vi "DV_Adjust_Histogram_Cursor.vi"(10 "lock to bin edges":bool, 11 "histogram reference":refnum<vi>) -> ()   [LabVIEW 2016]
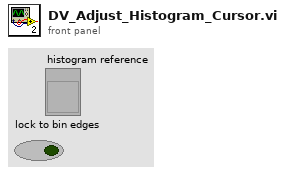
[diagram p1: front panel]
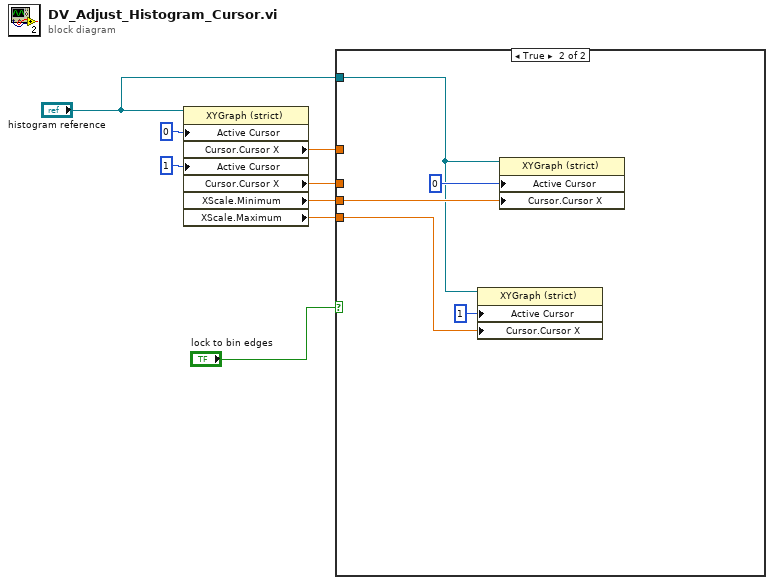
[diagram p0: block diagram]
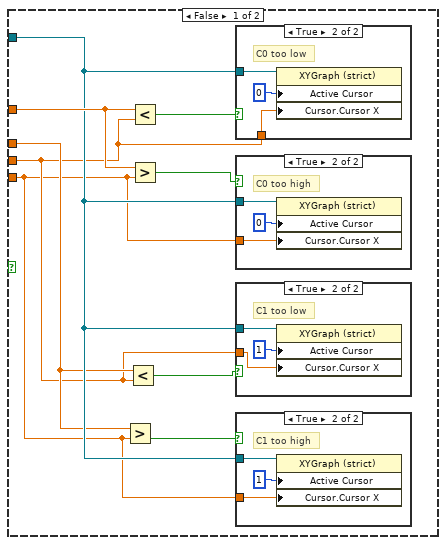
[diagram p2: hidden frame]
diagram:
  n1 = property on="Property Node" class="XYGraph (strict)"(reference="histogram reference", "Active Cursor"=0, "Active Cursor"=1) -> ("Cursor.Cursor X"=w6:dbl, "Cursor.Cursor X"=w4:dbl, "XScale.Minimum"=w3:dbl, "XScale.Maximum"=w2:dbl)  [unwired: 1 in, 2 out]
  n2 = case shown="True" "lock to bin edges" {
    tunnel: w6 -> [w16 _]
    tunnel: "histogram reference" -> [w14 w30]
    tunnel: w4 -> [w11 _]
    tunnel: w3 -> [w10 w33]
    tunnel: w2 -> [w9 w31]
    frame False {
      n3 = Greater?(x=w11, y=w9) -> (0:w12:bool)
      n4 = Less?(x=w11, y=w10) -> (x < y?=w13:bool)
      n5 = Less?(x=w16, y=w10) -> (x < y?=w17:bool)
      n6 = Greater?(x=w16, y=w9) -> (0:w15:bool)
      n7 = case shown="True" w17 {
        tunnel: w14 -> [_ w28]
        tunnel: w10 -> [_ w27]
        frame False {
        }
        frame True {
          # "C0 too low"
          n8 = property on="Property Node" class="XYGraph (strict)"(reference=w28, "Active Cursor"=0, "Cursor.Cursor X"=w27) -> ()  [unwired: 1 in, 2 out]
        }
      }
      n9 = case shown="True" w15 {
        tunnel: w14 -> [_ w25]
        tunnel: w9 -> [_ w24]
        frame False {
        }
        frame True {
          # "C0 too high"
          n10 = property on="Property Node" class="XYGraph (strict)"(reference=w25, "Active Cursor"=0, "Cursor.Cursor X"=w24) -> ()  [unwired: 1 in, 2 out]
        }
      }
      n11 = case shown="True" w13 {
        tunnel: w14 -> [_ w22]
        tunnel: w10 -> [_ w21]
        frame False {
        }
        frame True {
          # "C1 too low"
          n12 = property on="Property Node" class="XYGraph (strict)"(reference=w22, "Active Cursor"=1, "Cursor.Cursor X"=w21) -> ()  [unwired: 1 in, 2 out]
        }
      }
      n13 = case shown="True" w12 {
        tunnel: w14 -> [_ w19]
        tunnel: w9 -> [_ w18]
        frame False {
        }
        frame True {
          # "C1 too high"
          n14 = property on="Property Node" class="XYGraph (strict)"(reference=w19, "Active Cursor"=1, "Cursor.Cursor X"=w18) -> ()  [unwired: 1 in, 2 out]
        }
      }
    }
    frame True {
      n15 = property on="Property Node" class="XYGraph (strict)"(reference=w30, "Active Cursor"=1, "Cursor.Cursor X"=w31) -> ()  [unwired: 1 in, 2 out]
      n16 = property on="Property Node" class="XYGraph (strict)"(reference=w30, "Active Cursor"=0, "Cursor.Cursor X"=w33) -> ()  [unwired: 1 in, 2 out]
    }
  }
